vi "yzk3.2.vi"(1 "数值 2":dbl, 2 "数值":dbl, 3 "功能选择":enum16{"相减", "相乘", "相除", "相加"}(ring)) -> (0 "数值 3":dbl)   [LabVIEW 2017]
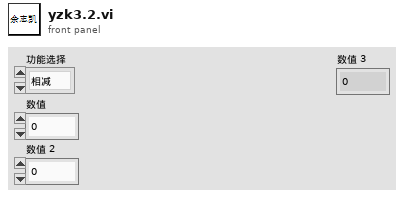
[diagram p1: front panel]
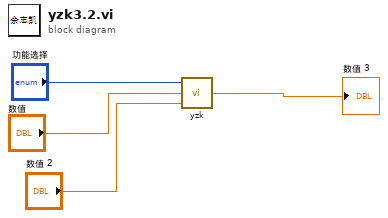
[diagram p0: block diagram]
diagram:
  n1 = call "yzk.vi"("数值 2"="数值 2", "数值"="数值", "功能选择"="功能选择") -> ("数值 3"=→"数值 3":dbl)
